vi "SignalRecovery7280Lock-inAmp.vi"() -> ()   [LabVIEW 2019]
uses:
  lib/Hardware/TextControlledInstrumIOQueuePacket.ctl
  lib/Hardware/TextControlledInstrum/TextControlledInstrumControlToCommandMulti.vi
panel:
  in  "Tab Control":T1(tab)
  in  "Connect":bool
  in  "Serial Port Setting":T2={"stop bits "=10, "flow control (0:none)"=0, "parity (none)"=enum."None", "data bits (8)"=8, "termination char (LF)"=10, "baud rate"=38400, "resource name"="COM4", "timeout (ms)"=500} {"baud rate" items=["110"=110, "300"=300, "600"=600, "1200"=1200, "2400"=2400, "4800"=4800, "9600"=9600, "19200"=19200, "38400"=38400, "57600"=57600, "115200"=115200, "230400"=230400, "460800"=460800, "921600"=921600, "1000000"=1000000, "2000000"=2000000, "4000000"=4000000]; "termination char (LF)" format="%02x"; "data bits (8)" min=5 max=8 step=1; "flow control (0:none)" items=["None", "XON/XOFF", "RTS/CTS", "XON/XOFF & RTS/CTS", "DTR/DSR", "XON/XOFF & DTR/DSR"]; "stop bits" items=["1.0"=10, "1.5"=15, "2.0"=20]}
  in  "Scale":dbl=1.0 min=0.0 format="%#.3p"
  out "X Scaled":dbl=5e-07 format="%#_6p"
  out "Y Scaled":dbl=-1.5e-06 format="%#_6p"
  out "Overload":bool
  out "Unlock":bool
  out "Status":u8 format="%02x"
  in  "Auto Phase":bool
  in  "Cluster":T3={"Voltage Input Mode"=0, "Input Shield Mode"=0, "Sensitivity"=20, "AC Gain"=5, "Automatic"=1, "Line Filter"=0, "Reference"=0, "Reference Source"=0, "Ref. Harmonic"=1, "Ref. Phase (degree)"=12.49, "Output Filter Slope"=1, "Time Constant"=15, "Synchronous Filter"=1, "Output Expansion"=0, "Output CH1"=0, "Output CH2"=1, "Oscillator Amp (Vrms)"=0.5, "Oscillator Freq (Hz)"=1200.0} {"Oscillator Freq (Hz)" min=0.0 max=2000000.0 format="%#_6p"; "Oscillator Amp (Vrms)" min=0.0 max=1.0 step=0.001 format="%#.3f"; "Output CH2" items=["X % (2.5 V FS)", "Y % (2.5 V FS)", "R % (2.5 V FS)", "Phase (30 deg/V, 0V=0deg)", "Phase (30 deg/V, -9V=0deg)", "Noise % (2.5 V FS)", "Raitio (10 x X%/ADC 1)", "Ratio log10(10 x X%/ADC1)", "Equation 1", "Equation 2", "X2 % (2.5 V FS)", "Y2 % (2.5 V FS)", "R2 % (2.5 V FS)", "Phase2 (30 deg/V, 0V=0deg)", "Phase2 (30 deg/V, -9V=0deg)"]; "Output CH1" items=["X % (2.5 V FS)", "Y % (2.5 V FS)", "R % (2.5 V FS)", "Phase (30 deg/V, 0V=0deg)", "Phase (30 deg/V, -9V=0deg)", "Noise % (2.5 V FS)", "Raitio (10 x X%/ADC 1)", "Ratio log10(10 x X%/ADC1)", "Equation 1", "Equation 2", "X2 % (2.5 V FS)", "Y2 % (2.5 V FS)", "R2 % (2.5 V FS)", "Phase2 (30 deg/V, 0V=0deg)", "Phase2 (30 deg/V, -9V=0deg)"]; "Output Expansion" items=["Off", "Expand X", "Expand Y", "Expand X & Y"]; "Synchronous Filter" items=["Disabled", "Enabled"]; "Time Constant" items=["500 us"=8, "1 ms"=9, "2 ms"=10, "5 ms"=11, "10 ms"=12, "20 ms"=13, "50 ms"=14, "100 ms"=15, "200 ms"=16, "500 ms"=17, "1 s"=18, "2 s"=19, "5 s"=20, "10 s"=21, "20 s"=22, "50 s"=23, "100 s"=24, "200 s"=25, "500 s"=26, "1 ks"=27, "2 ks"=28, "5 ks"=29, "10 ks"=30, "20 ks"=31, "50 ks"=32, "100 ks"=33, ""=34]; "Output Filter Slope" items=["6 dB/oct", "12 dB/oct", "18 dB/oct (TC>=0.5ms)", "24 dB/oct (TC>=0.5ms)"]; "Ref. Phase (degree)" min=0.0 max=360.0 step=90.0 format="%#.3f"; "Ref. Harmonic" min=1 max=32 step=1; "Reference Source" items=["Internal", "Ext. Logic", "Ext. Analog"]; "Reference" items=["Single / Virtual", "Dual Harmonic", "Dual Reference"]; "Line Filter" items=["Off", "50 Hz", "100 Hz", "50 Hz & 100 Hz"]; "Automatic" items=["No", "Yes"]; "AC Gain" items=["0 dB", "6 dB", "14 dB", "20 dB", "26 dB", "34 dB", "40 dB", "46 dB", "54 dB", "60 dB", "66 dB"]; "Sensitivity" items=["10 nV"=3, "20 nV"=4, "50 nV"=5, "100 nV"=6, "200 nV"=7, "500 nV"=8, "1 uV"=9, "2 uV"=10, "5 uV"=11, "10 uV"=12, "20 uV"=13, "50 uV"=14, "100 uV"=15, "200 uV"=16, "500 uV"=17, "1 mV"=18, "2 mV"=19, "5 mV"=20, "10 mV"=21, "20 mV"=22, "50 mV"=23, "100 mV"=24, "200 mV"=25, "500 mV"=26, "1 V"=27]; "Input Shield Mode" items=["Ground", "Float (1kOhm to GND)"]; "Voltage Input Mode" items=["Both inputs grounded", "A input only", "-B input only", "A-B differential"]}
  out "Serial Port":refnum<visa-resource-name>="COM4"
  out "Frequency":dbl=1200.0 min=0.0 max=360.0 step=0.001 format="%#.3p"
  out "X":dbl=5e-07 format="%#_6p"
  out "Y":dbl=-1.5e-06 format="%#_6p"
  # "resource name で COM ポートを指定したら\nSIGNAL RECOVERY 7280 タブを選択すれば繋がる"
  # "Lock-in Amp とシリアル通信するにはクロスケーブルが必要\nAUX ではない方に繋ぐ\n\nLock-in Amp 側の Menu-Configuration-\nCommunications-RS232 settings メニューで\n以下を設定しておく\n  Baud Rate = 38400\n  Data Bits = 8\n  Parity = none\n  Echo = on\n  Prompt = on\n  Delimiter = , (ASCII 44)"
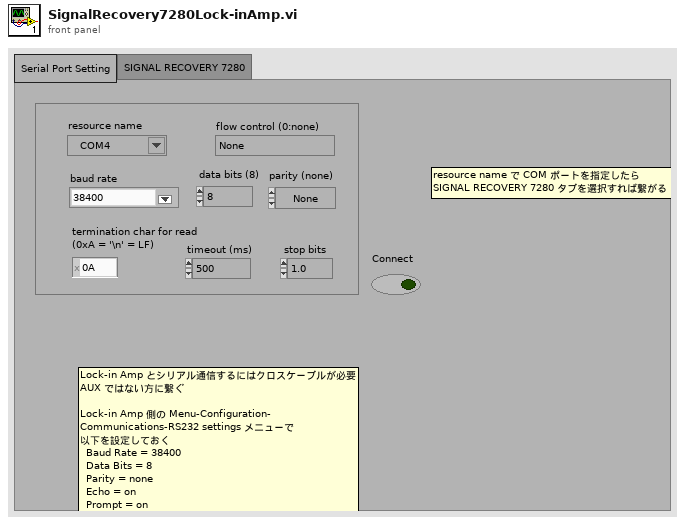
[diagram p1: front panel]
types:
  T1 = enum32{"Serial Port Setting", "SIGNAL RECOVERY 7280"}
  T2 = cluster{"stop bits ":u16, "flow control (0:none)":u16, "parity (none)":enum16{"None", "Odd", "Even", "Mark", "Space"}, "data bits (8)":u16, "termination char (LF)":u8, "baud rate":u32, "resource name":refnum<visa-resource-name>, "timeout (ms)":u32}
  T3 = cluster{"Voltage Input Mode":u16, "Input Shield Mode":u16, "Sensitivity":u16, "AC Gain":u16, "Automatic":u16, "Line Filter":u16, "Reference":u16, "Reference Source":u16, "Ref. Harmonic":u32, "Ref. Phase (degree)":dbl, "Output Filter Slope":u16, "Time Constant":u16, "Synchronous Filter":u16, "Output Expansion":u16, "Output CH1":u16, "Output CH2":u16, "Oscillator Amp (Vrms)":dbl, "Oscillator Freq (Hz)":dbl}
  T4 = typedef "TextControlledInstrumIOQueuePacket.ctl" = cluster{"Operation":enum16{"read", "write", "reserved2", "reserved3", "reserved4", "reserved5", "reserved6", "reserved7"}, "Data":string, "Queue":refnum<queue>}
  T5 = enum16{"read", "write", "reserved2", "reserved3", "reserved4", "reserved5", "reserved6", "reserved7"}
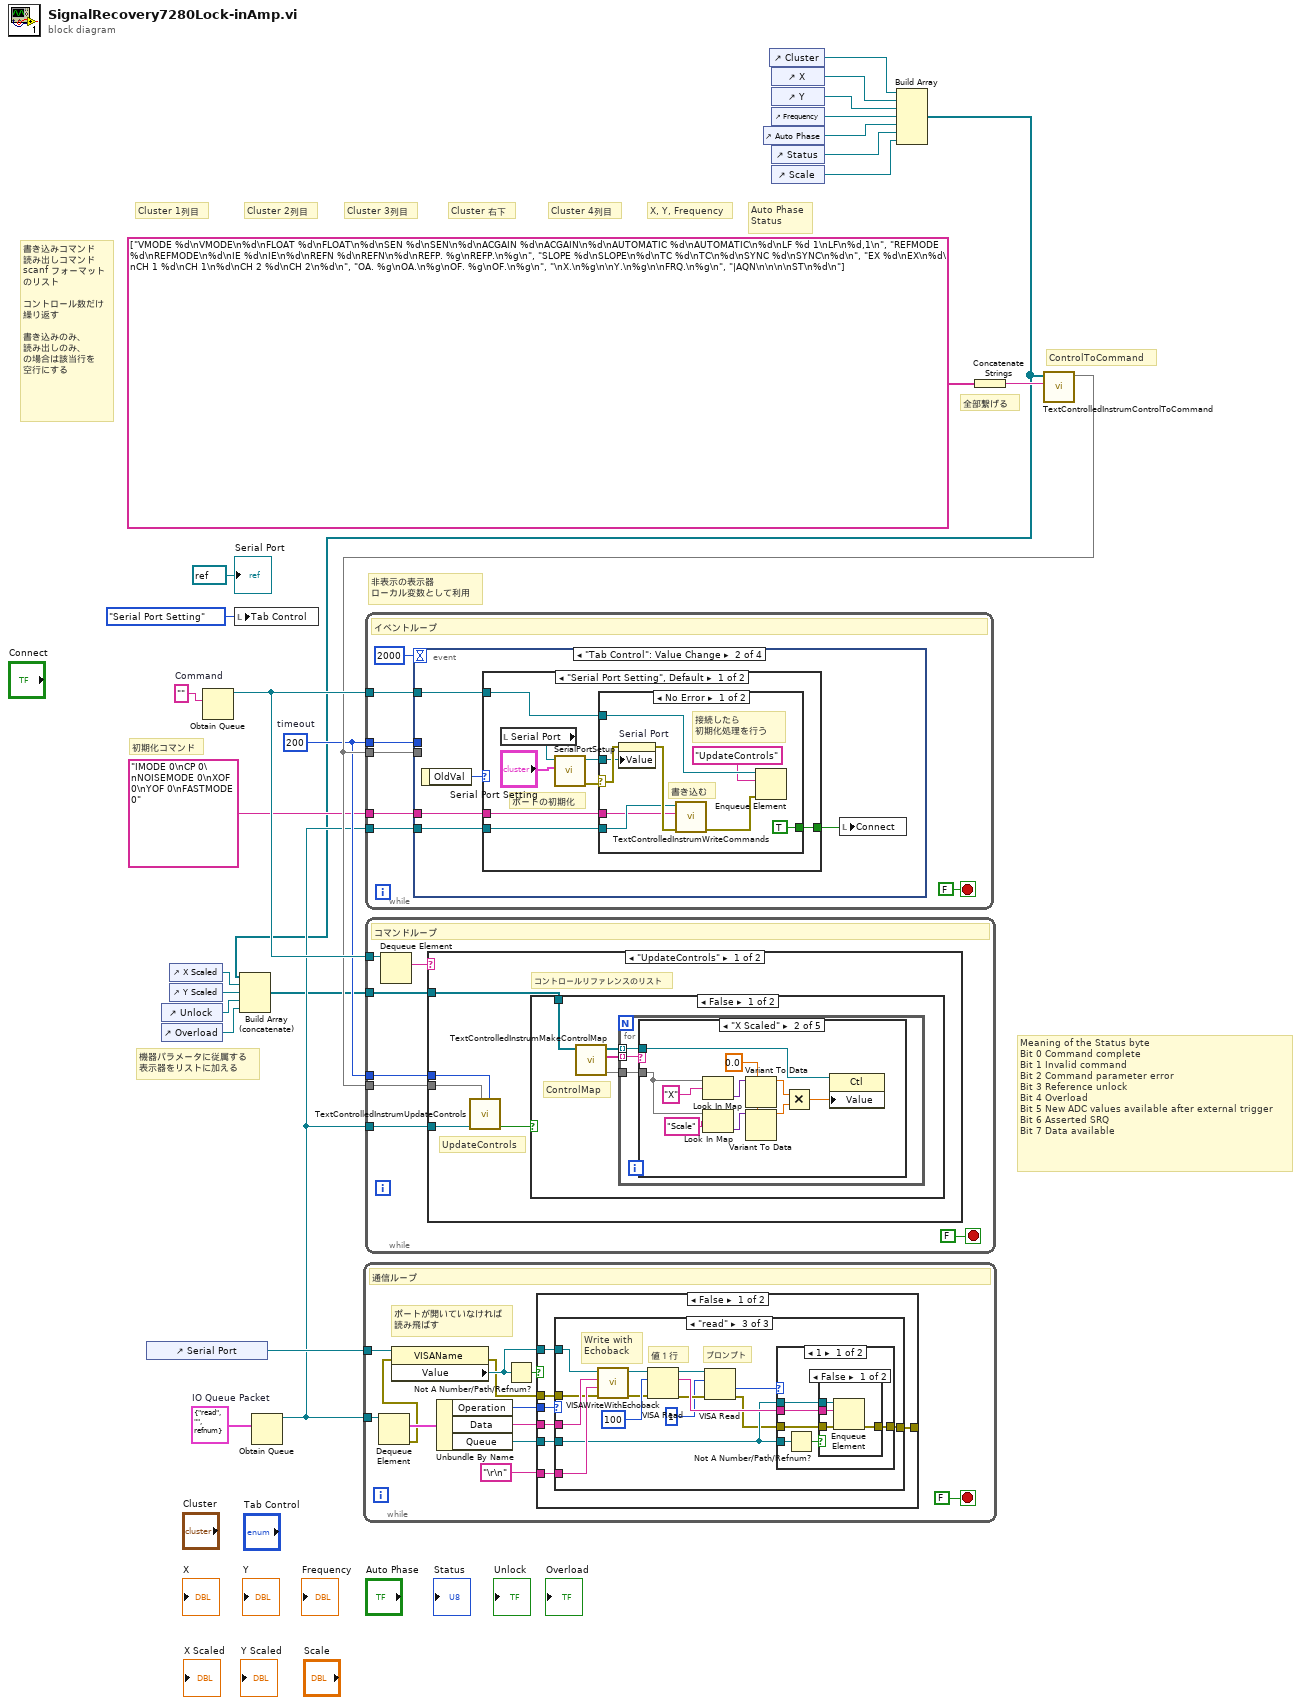
[diagram p0: block diagram]
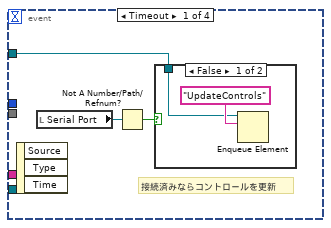
[diagram p2: hidden frame]
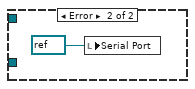
[diagram p4: hidden frame]
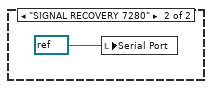
[diagram p5: hidden frame]
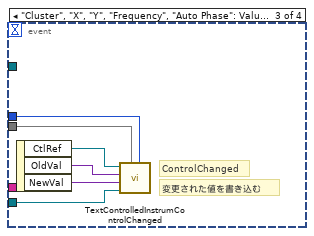
[diagram p6: hidden frame]
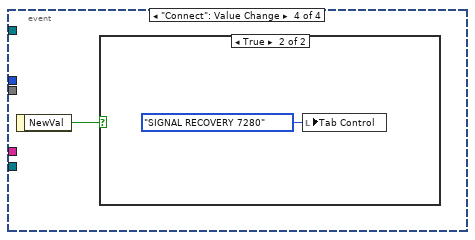
[diagram p7: hidden frame]
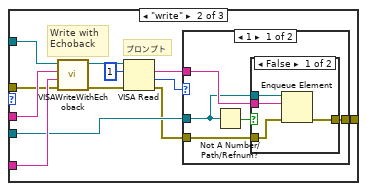
[diagram p10: hidden frame]
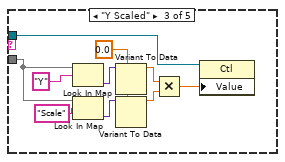
[diagram p17: hidden frame]
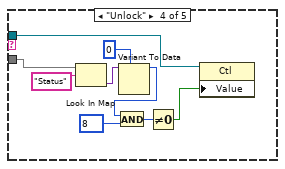
[diagram p18: hidden frame]
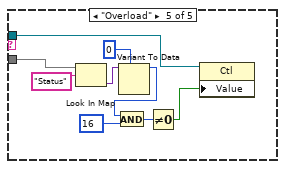
[diagram p19: hidden frame]
diagram:
  w13 = ""  # Command
  w22 = T4 {"Operation"=enum."read", "Data"="", "Queue"=refnum}  # IO Queue Packet
  w10 = 200  # timeout
  # "機器パラメータに従属する\n表示器をリストに加える"
  # "非表示の表示器\nローカル変数として利用"
  # "Meaning of the Status byte\nBit 0 Command complete\nBit 1 Invalid command\nBit 2 Command parameter error\nBit 3 Reference unlock\nBit 4 Overload\nBit 5 New ADC values available after external trigger\nBit 6 Asserted SRQ\nBit 7 Data available"
  # "ControlToCommand"
  # "全部繋げる"
  # "Auto Phase\nStatus"
  # "X, Y, Frequency"
  # "Cluster 4列目"
  # "Cluster 右下"
  # "Cluster 3列目"
  # "Cluster 2列目"
  # "Cluster 1列目"
  # "初期化コマンド"
  # "書き込みコマンド\n読み出しコマンド\nscanf フォーマット\nのリスト\n\nコントロール数だけ\n繰り返す\n\n書き込みのみ、\n読み出しのみ、\nの場合は該当行を\n空行にする"
  n1 = control-ref of="Serial Port"() -> (w17:refnum<vi>)
  n2 = control-ref of="Unlock"() -> (w5:refnum<vi>)
  n3 = control-ref of="Overload"() -> (w4:refnum<vi>)
  n4 = control-ref of="X Scaled"() -> (w3:refnum<vi>)
  n5 = control-ref of="Y Scaled"() -> (w6:refnum<vi>)
  n6 = Obtain Queue(element data type=w13) -> (queue out=w12:refnum<queue>)  [unwired: 4 in, 2 out]
  n7 = local write "Tab Control"(T1."Serial Port Setting" ("Tab Control")) -> ()
  n8 = Obtain Queue(element data type=w22) -> (queue out=w9:refnum<queue>)  [unwired: 4 in, 2 out]
  n9 = while {
    tunnel: w9 -> [w35]
    tunnel: w17 -> [w34]
    stop <- FALSE stop-if-true
    # "ポートが開いていなければ\n読み飛ばす"
    # "通信ループ"
    n10 = Dequeue Element(queue=w35) -> (element=w36:T4, error out=w27:errorcluster)  [unwired: 2 in, 2 out]
    n11 = property class="VISAName"(reference=w34, error in=w27) -> (error out=w26:errorcluster, "Value"=w28:refnum<visa-resource-name>)  [unwired: 1 out]
    n12 = Unbundle By Name(w36) -> ("Operation"=w32:T5, "Data"=w30:string, "Queue"=w31:refnum<queue>)
    n13 = Not A Number/Path/Refnum?(number/path/refnum=w28) -> (NaN/Path/Refnum?=w33:bool)
    n14 = case shown="False" w33 {
      tunnel: w32 -> [w44 _]
      tunnel: w28 -> [w43 _]
      tunnel: w30 -> [w42 _]
      tunnel: w31 -> [w41 _]
      tunnel: "\r\n" -> [w40 _]
      tunnel: w26 -> [w39 w96]
      tunnel: [w38 w96] -> _
      frame False {
        n15 = case shown="\"read\"" w44 {
          tunnel: w43 -> [_ w57 w81]
          tunnel: w42 -> [_ w56 w80]
          tunnel: w41 -> [_ w51 w72]
          tunnel: w40 -> [_ w55 w79]
          tunnel: w39 -> [w45 w48 w71]
          tunnel: [w45 w46 w69] -> w38
          frame Default {
          }
          frame "write" {
            # "Write with \nEchoback"
            # "プロンプト"
            n16 = call "VISAWriteWithEchoback.vi"("error in"=w48, "termination"=w55, "write data"=w56, "VISA resource name"=w57) -> ("error out"=w50:errorcluster, "VISA resource name out"=w54:refnum<visa-resource-name>)  [unwired: 5 in, 1 out]
            n17 = VISA Read(VISA resource name=w54, byte count=u32 1, error in (no error)=w50) -> (read buffer=w52:string, return count=w49:u32, error out=w47:errorcluster)  [unwired: 1 out]
            n18 = case shown="1" w49 {
              tunnel: w52 -> [w62 _]
              tunnel: w51 -> [w61 _]
              tunnel: w47 -> [w59 w68]
              tunnel: [w58 w68] -> w46
              frame 1 {
                n19 = Not A Number/Path/Refnum?(number/path/refnum=w61) -> (NaN/Path/Refnum?=w60:bool)
                n20 = case shown="False" w60 {
                  tunnel: w62 -> [w66 _]
                  tunnel: w61 -> [w65 _]
                  tunnel: w59 -> [w64 w67]
                  tunnel: [w63 w67] -> w58
                  frame False {
                    n21 = Enqueue Element(queue=w65, element=w66, error in (no error)=w64) -> (error out=w63:errorcluster)  [unwired: 1 in, 2 out]
                  }
                  frame True {
                  }
                }
              }
              frame Default {
              }
            }
          }
          frame "read" {
            # "プロンプト"
            # "値１行"
            # "Write with \nEchoback"
            n22 = call "VISAWriteWithEchoback.vi"("error in"=w71, "termination"=w79, "write data"=w80, "VISA resource name"=w81) -> ("error out"=w77:errorcluster, "VISA resource name out"=w78:refnum<visa-resource-name>)  [unwired: 5 in, 1 out]
            n23 = VISA Read(VISA resource name=w78, byte count=u32 100, error in (no error)=w77) -> (VISA resource name out=w76:refnum<visa-resource-name>, read buffer=w82:string, error out=w75:errorcluster)  [unwired: 1 out]
            n24 = VISA Read(VISA resource name=w76, byte count=u32 1, error in (no error)=w75) -> (return count=w73:u32, error out=w70:errorcluster)  [unwired: 2 out]
            n25 = case shown="1" w73 {
              tunnel: w72 -> [w89 _]
              tunnel: w82 -> [w88 _]
              tunnel: w72 -> [w87 _]
              tunnel: w70 -> [w85 w95]
              tunnel: [w84 w95] -> w69
              frame 1 {
                n26 = Not A Number/Path/Refnum?(number/path/refnum=w87) -> (NaN/Path/Refnum?=w86:bool)
                n27 = case shown="False" w86 {
                  tunnel: w89 -> [w93 _]
                  tunnel: w88 -> [w92 _]
                  tunnel: w85 -> [w91 w94]
                  tunnel: [w90 w94] -> w84
                  frame False {
                    n28 = Enqueue Element(queue=w93, element=w92, error in (no error)=w91) -> (error out=w90:errorcluster)  [unwired: 1 in, 2 out]
                  }
                  frame True {
                  }
                }
              }
              frame Default {
              }
            }
          }
        }
      }
      frame True {
      }
    }
  }
  n29 = control-ref of="Auto Phase"() -> (w18:refnum<vi>)
  n30 = control-ref of="Cluster"() -> (w23:refnum<vi>)
  n31 = control-ref of="X"() -> (w21:refnum<vi>)
  n32 = control-ref of="Y"() -> (w20:refnum<vi>)
  n33 = control-ref of="Frequency"() -> (w19:refnum<vi>)
  n34 = control-ref of="Status"() -> (w14:refnum<vi>)
  n35 = control-ref of="Scale"() -> (w7:refnum<vi>)
  n36 = Build Array(w23, w21, w20, w19, w18, w14, w7) -> (w1:refnum<vi>[])
  n37 = Build Array (concatenate)(w1, w3, w6, w5, w4) -> (w2:refnum<vi>[])
  n38 = Concatenate Strings(string[] ["VMODE %d\nVMODE\n%d\nFLOAT %d\nFLOAT\n%d\nSEN %d\nSEN\n%d\nACGAIN %d\nACGAIN\n%d\nAUTOMATIC %d\nAUTOMATIC\n%d\nLF %d 1\nLF\n%d,1\n", "REFMODE %d\nREFMODE\n%d\nIE %d\nIE\n%d\nREFN %d\nREFN\n%d\nREFP. %g\nREFP.\n%g\n", "SLOPE %d\nSLOPE\n%d\nTC %d\nTC\n%d\nSYNC %d\nSYNC\n%d\n", "EX %d\nEX\n%d\nCH 1 %d\nCH 1\n%d\nCH 2 %d\nCH 2\n%d\n", "OA. %g\nOA.\n%g\nOF. %g\nOF.\n%g\n", "\nX.\n%g\n\nY.\n%g\n\nFRQ.\n%g\n", "|AQN\n\n\n\nST\n%d\n"]) -> (w15:string)
  n39 = call-poly "TextControlledInstrumControlToCommand.vi"("SetGetCommands"=w15, "Control Array"=w1) -> ("ControlToCommand"=w11:map{refnum<vi>, string[]})  [unwired: 9 in]
  n40 = while {
    tunnel: w11 -> [w101]
    tunnel: w9 -> [w100]
    tunnel: w10 -> [w99]
    tunnel: w12 -> [w98]
    tunnel: "IMODE 0\nCP 0\nNOISEMODE 0\nXOF 0\nYOF 0\nFASTMODE 0" -> [w97]
    stop <- FALSE stop-if-true
    # "イベントループ"
    n41 = event shown="[1] \"Tab Control\": Value Change" {
      selector: _ -> [_ _ _ _]
      dyn-events: _ -> [_ _ _ _]
      timeout: 2000 -> [_ _ _ _]
      tunnel: w101 -> [_ _ w133 _]
      tunnel: w100 -> [_ w112 w134 _]
      tunnel: w99 -> [_ _ w135 _]
      tunnel: w98 -> [w106 w111 _ _]
      tunnel: w97 -> [_ w110 _ _]
      event Timeout {
        # "接続済みならコントロールを更新"
        n42 = event-data() -> ()  [unwired: 1 in, 3 out]
        n43 = local read "Serial Port"() -> (w105:refnum<visa-resource-name>)
        n44 = Not A Number/Path/Refnum?(number/path/refnum=w105) -> (NaN/Path/Refnum?=w104:bool)
        n45 = case shown="False" w104 {
          tunnel: w106 -> [w107 _]
          frame False {
            n46 = Enqueue Element(queue=w107, element="UpdateControls") -> ()  [unwired: 2 in, 3 out]
          }
          frame True {
          }
        }
      }
      event "Tab Control": Value Change {
        n47 = event-data() -> ("OldVal"=w113:T1)  [unwired: 1 in]
        n48 = case shown="\"Serial Port Setting\", Default" w113 {
          tunnel: w112 -> [w117 _]
          tunnel: w111 -> [w116 _]
          tunnel: w110 -> [w115 _]
          tunnel: [w114 _] -> w109
          frame "Serial Port Setting", Default {
            # "ポートの初期化"
            n49 = local read "Serial Port"() -> (w121:refnum<visa-resource-name>)
            n50 = call "SerialPortSetup.vi"("Serial Port Setting"="Serial Port Setting", "VISA resource name (will be closed)"=w121) -> ("error out"=w119:errorcluster, "VISA resource name out"=w118:refnum<visa-resource-name>)  [unwired: 8 in]
            n51 = case shown="No Error" w119 {
              selector: w119 -> [w130 _]
              tunnel: w118 -> [w129 _]
              tunnel: w117 -> [w127 _]
              tunnel: w116 -> [w126 _]
              tunnel: w115 -> [w123 _]
              tunnel: [TRUE _] -> w114
              frame No Error {
                # "接続したら\n初期化処理を行う"
                # "書き込む"
                n52 = property on="Serial Port" class="VISAName"(error in=w130, "Value"=w129) -> (error out=w128:errorcluster)  [unwired: 1 in, 1 out]
                n53 = call "TextControlledInstrumWriteCommands.vi"("error in (no error)"=w128, "Multi-line String"=w123, "IO Queue"=w127) -> ("error out"=w124:errorcluster)  [unwired: 7 in, 1 out]
                n54 = Enqueue Element(queue=w126, element="UpdateControls", error in (no error)=w124) -> ()  [unwired: 1 in, 3 out]
              }
              frame Error {
                n55 = local write "Serial Port"(refnum<visa-resource-name> refnum ("t")) -> ()
              }
            }
          }
          frame "SIGNAL RECOVERY 7280" {
            n56 = local write "Serial Port"(refnum<visa-resource-name> refnum ("t")) -> ()
          }
        }
        n57 = local write "Connect"(w109) -> ()
      }
      event "Cluster", "X", "Y", "Frequency", "Auto Phase": Value Change {
        # "ControlChanged"
        # "変更された値を書き込む"
        n58 = event-data() -> ("CtlRef"=w138:refnum<vi>, "OldVal"=w137:variant, "NewVal"=w136:variant)  [unwired: 1 in]
        n59 = call "TextControlledInstrumControlChanged.vi"("timeout in ms (1000ms)"=w135, "ControlToCommand"=w133, "IO Queue"=w134, "NewVal"=w136, "OldVal"=w137, "CtlRef"=w138) -> ()  [unwired: 5 in, 1 out]
      }
      event "Connect": Value Change {
        n60 = event-data() -> ("NewVal"=w139:bool)  [unwired: 1 in]
        n61 = case shown="True" w139 {
          frame False {
          }
          frame True {
            n62 = local write "Tab Control"(T1."SIGNAL RECOVERY 7280" ("Tab Control")) -> ()
          }
        }
      }
    }
  }
  n63 = while {
    tunnel: w12 -> [w146]
    tunnel: w11 -> [w144]
    tunnel: w10 -> [w143]
    tunnel: w9 -> [w142]
    tunnel: w2 -> [w141]
    stop <- FALSE stop-if-true
    # "コマンドループ"
    n64 = Dequeue Element(queue=w146) -> (element=w147:string)  [unwired: 2 in, 3 out]
    n65 = case shown="\"UpdateControls\"" w147 {
      tunnel: w143 -> [w152 _]
      tunnel: w142 -> [w149 _]
      tunnel: w144 -> [w150 _]
      tunnel: w141 -> [w151 _]
      frame "UpdateControls" {
        # "コントロールリファレンスのリスト"
        # "UpdateControls"
        n66 = call "TextControlledInstrumUpdateControls.vi"("timeout in ms (1000ms)"=w152, "ControlToCommand"=w150, "IO Queue"=w149) -> ("timed out?"=w148:bool)  [unwired: 8 in]
        n67 = case shown="False" w148 {
          tunnel: w151 -> [w156 _]
          frame False {
            # "ControlMap"
            n68 = call "TextControlledInstrumMakeControlMap.vi"("ControlArray"=w156) -> ("ValueMap out"=w153:map{string, variant}, "Names"=w155:string[], "Controls"=w154:refnum<vi>[])  [unwired: 7 in, 1 out]
            n69 = for {
              tunnel: w155 -> [w159] mode=indexing
              tunnel: w153 -> [w158]
              tunnel: w154 -> [w157] mode=indexing
              n70 = case shown="\"X Scaled\"" w159 {
                tunnel: w158 -> [_ w167 w177 w187 w196]
                tunnel: w157 -> [_ w161 w171 w184 w193]
                frame Default {
                }
                frame "X Scaled" {
                  w164 = 0.0
                  n71 = Look In Map(map=w167, key="X") -> (value=w166:variant)  [unwired: 1 in, 1 out]
                  n72 = Look In Map(map=w167, key="Scale") -> (value=w165:variant)  [unwired: 1 in, 1 out]
                  n73 = Variant To Data(type=w164, Variant=w166) -> (data=w163:dbl)  [unwired: 1 in, 1 out]
                  n74 = Variant To Data(type=w164, Variant=w165) -> (data=w162:dbl)  [unwired: 1 in, 1 out]
                  n75 = Multiply(x=w163, y=w162) -> (x*y=w160:dbl)
                  n76 = property class="Ctl"(reference=w161, "Value"=w160) -> ()  [unwired: 1 in, 2 out]
                }
                frame "Y Scaled" {
                  w174 = 0.0
                  n77 = Look In Map(map=w177, key="Y") -> (value=w176:variant)  [unwired: 1 in, 1 out]
                  n78 = Look In Map(map=w177, key="Scale") -> (value=w175:variant)  [unwired: 1 in, 1 out]
                  n79 = Variant To Data(type=w174, Variant=w176) -> (data=w173:dbl)  [unwired: 1 in, 1 out]
                  n80 = Variant To Data(type=w174, Variant=w175) -> (data=w172:dbl)  [unwired: 1 in, 1 out]
                  n81 = Multiply(x=w173, y=w172) -> (x*y=w170:dbl)
                  n82 = property class="Ctl"(reference=w171, "Value"=w170) -> ()  [unwired: 1 in, 2 out]
                }
                frame "Unlock" {
                  n83 = Look In Map(map=w187, key="Status") -> (value=w186:variant)  [unwired: 1 in, 1 out]
                  n84 = Variant To Data(type=u8 0, Variant=w186) -> (data=w183:u8)  [unwired: 1 in, 1 out]
                  n85 = And(x=w183, y=u8 8) -> (x .and. y?=w181:u8)
                  n86 = Not Equal To 0?(x=w181) -> (x != 0?=w180:bool)
                  n87 = property class="Ctl"(reference=w184, "Value"=w180) -> ()  [unwired: 1 in, 2 out]
                }
                frame "Overload" {
                  n88 = Look In Map(map=w196, key="Status") -> (value=w195:variant)  [unwired: 1 in, 1 out]
                  n89 = Variant To Data(type=u8 0, Variant=w195) -> (data=w192:u8)  [unwired: 1 in, 1 out]
                  n90 = And(x=w192, y=u8 16) -> (x .and. y?=w190:u8)
                  n91 = Not Equal To 0?(x=w190) -> (x != 0?=w189:bool)
                  n92 = property class="Ctl"(reference=w193, "Value"=w189) -> ()  [unwired: 1 in, 2 out]
                }
              }
            }
          }
          frame True {
          }
        }
      }
      frame Default {
      }
    }
  }
  "Serial Port" <- refnum<visa-resource-name> refnum ("t")
